vi "Untitled 1.vi"   [LabVIEW 2016]
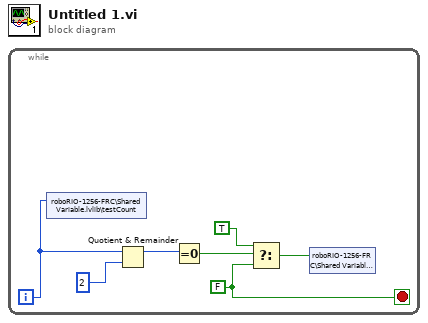
[diagram p0: block diagram]
diagram:
  n1 = while {
    i -> [w1]
    stop <- w2 stop-if-true
    w2 = FALSE
    n2 = shared-variable "roboRIO-1256-FRC\\Shared Variable.lvlib\\testCount"(w1) -> ()  [unwired: 1 in, 1 out]
    n3 = Quotient & Remainder(x=w1, y=2) -> (x-y*floor(x/y)=w6:i32)  [unwired: 1 out]
    n4 = Equal To 0?(x=w6) -> (x = 0?=w5:bool)
    n5 = Select(t=TRUE, s=w5, f=w2) -> (s? t:f=w4:bool)
    n6 = shared-variable "roboRIO-1256-FRC\\Shared Variable.lvlib\\test"(w4) -> ()  [unwired: 1 in, 1 out]
  }
